vi "ecg_ncs_v1c.vi"() -> ()   [LabVIEW 2016]
uses:
  <instrlib>/niUSRP/niUSRP Timestamp.ctl
  C:/Program Files/National Instruments/LabVIEW 2016/examples/Instrument IO/Serial/support/Serial - Settings.ctl
  <vilib>/Analysis/coordinate.llb/Wrap Angle (array).vi
  <instrlib>/niUSRP/niUSRP Configure Time Start Trigger.vi
  <vilib>/Instr/_visa.llb/VISA Configure Serial Port (Instr).vi
  <instrlib>/niUSRP/niUSRP Write Tx Data (2D CDB).vi
  <instrlib>/niUSRP/niUSRP Fetch Rx Data (2D CDB).vi
  <vilib>/Analysis/3filter.llb/Butterworth Filter (DBL).vi
  <vilib>/measure/NI_MABase.lvlib
  <vilib>/Analysis/NI_AALBase.lvlib
  <vilib>/Analysis/NI_AALPro.lvlib
  <vilib>/Analysis/NI_AAL_Angle.lvlib
panel:
  out "Poor Sensor Quality: \nSensor off":bool
  out "Poor Sensor Quality: \nSensor on":bool
  out "Heart Rate 2":u16[](array[numeric])
  out "Stop Loop":bool
  out "Loop index":i32
  out "size(s)":i32
  in  "Read Count":u32=960
  out "return count":u32
  out "Serial Settings:Number of Bytes at Serial Port":u32
  in  "Serial Settings":T1={"baud rate"=57600, "data bits"=8, "parity"=enum."None", "stop bits"=10, "flow control"=0} {"flow control" items=["None"=0, "XON/XOFF"=1, "RTS/CTS"=2, "DTR/DSR"=4]; "stop bits" items=["1.0"=10, "1.5"=15, "2.0"=20]; "data bits" min=5 max=8 step=1; "baud rate" items=["75"=75, "110"=110, "134"=134, "150"=150, "300"=300, "600"=600, "1200"=1200, "1800"=1800, "2400"=2400, "4800"=4800, "7200"=7200, "9600"=9600, "14400"=14400, "19200"=19200, "28800"=28800, "38400"=38400, "56000"=56000, "57600"=57600, "115200"=115200, "128000"=128000, "230400"=230400]}
  in  "VISA resource name":refnum<visa-resource-name>="bmd101"
  in  "?":enum32{"ECG", "Heart Rate"}(tab)
  out "ECG":i16(graph)
  out "Heart Rate":u8[](graph)
  in  "Stop":bool
  in  "File Name":string="Test"
  in  "order1":i32=5
  in  "Path":path=path "D:/Research/SummerFall17Spring18/CnC/NCS/EcgNcsCorrelation"
  in  "Low-Pass Freq":dbl=200.0 format="%#_13g"
  in  "Sampling Rate":i32=500
  out "Gain":dbl=-15.0
  out "Bandwidth":dbl=56000000.0
  out "Coerced Carrier Frequency":dbl=2000000000.0 format="%#.17g"
  out "Coerced Tx IQ rate":dbl=1000000.0
  out "Coerced Rx IQ rate":dbl=1000000.0
  out "error IO":errorcluster={"status"=FALSE, "code"=-1074118647, "source"=""}
  in  "Rx Number of Samples":i32=20000
  in  "Tab Control 2":enum32{"NI-294x/295x", "NI-2900/2901"}(tab)=enum."NI-2900/2901"
  in  "channel 0 carrier\n frequency [Hz]":dbl=2000000000.0 format="%#_6p"
  in  "Rx carrier frequency [Hz]":dbl=2000000000.0 format="%#_6p"
  in  "Tx carrier frequency [Hz]":dbl=1000000000.0 format="%#_6p"
  in  "Start Trigger Time":T2={"whole seconds"=1, "fractional seconds"=0.0}
  out "Tx Active Antenna":string="TX1"
  in  "Tab Control":T3(tab)
  out "NCS tag Amp":dbl[](graph)=[0.013332788438327721, 0.0131552898712497, 0.012994905519721597, 0.012986271887777701, 0.013075284595455733, 0.013191204808537919, 0.013351894528100879, 0.01345386740636616, 0.013382234051438232, 0.013180163786137358]
  out "NCS tag Phase":dbl[](graph)=[114.08993023907641, 111.82225141412982, 110.02998222947944, 109.41153055749608, 110.12587965469353, 112.16042160734105, 113.81215100166591, 114.51260226782536, 113.6206368361215, 111.46787264294511]
  out "IQ":dbl[][](graph)
  out "Tag Amp":dbl[](graph)
  out "Tag Phase":dbl[](graph)
  out "Tx Waveform Graph":waveform(dbl)[](graph)=[{"t0"=timestamp(0 s since 1904-01-01), "dt"=1e-06, "Y"=array[2000 elements]}, {"t0"=timestamp(0 s since 1904-01-01), "dt"=1e-06, "Y"=array[2000 elements]}]
  in  "Channel 0\nTone Amplitude":dbl=0.707 step=0.05 format="%#.6g"
  in  "Channel 0 \nTone Frequency":dbl=5000.0 format="%#_6p"
  in  "Waveform Size":dbl=2000.0
  in  "Rx Active Antenna":string="RX2"
  in  "Device Name":refnum<k15>="MyB200"
  in  "Tx Gain":dbl=28.0 format="%#_6f"
  in  "Tx IQ Rate":dbl=1000000.0 format="%#_6p"
  in  "Rx Gain":dbl=32.0 format="%#_6f"
  in  "Rx IQ Rate":dbl=1000000.0 format="%#_6p"
  # "Rx Settings"
  # "Tx Settings"
  # "Note that on the NI-2900 and NI-2901, both Rx channels share an LO and both Tx channels share an LO. However, on the NI-294x/295x devices, Rx and Tx of channel 0 share an LO and Rx and Tx of channel 1 share an LO."
  # "This Tx graph should always have end and start tied up since this is being sent in a loop continuously. Otherwise phase jumps will be noticed."
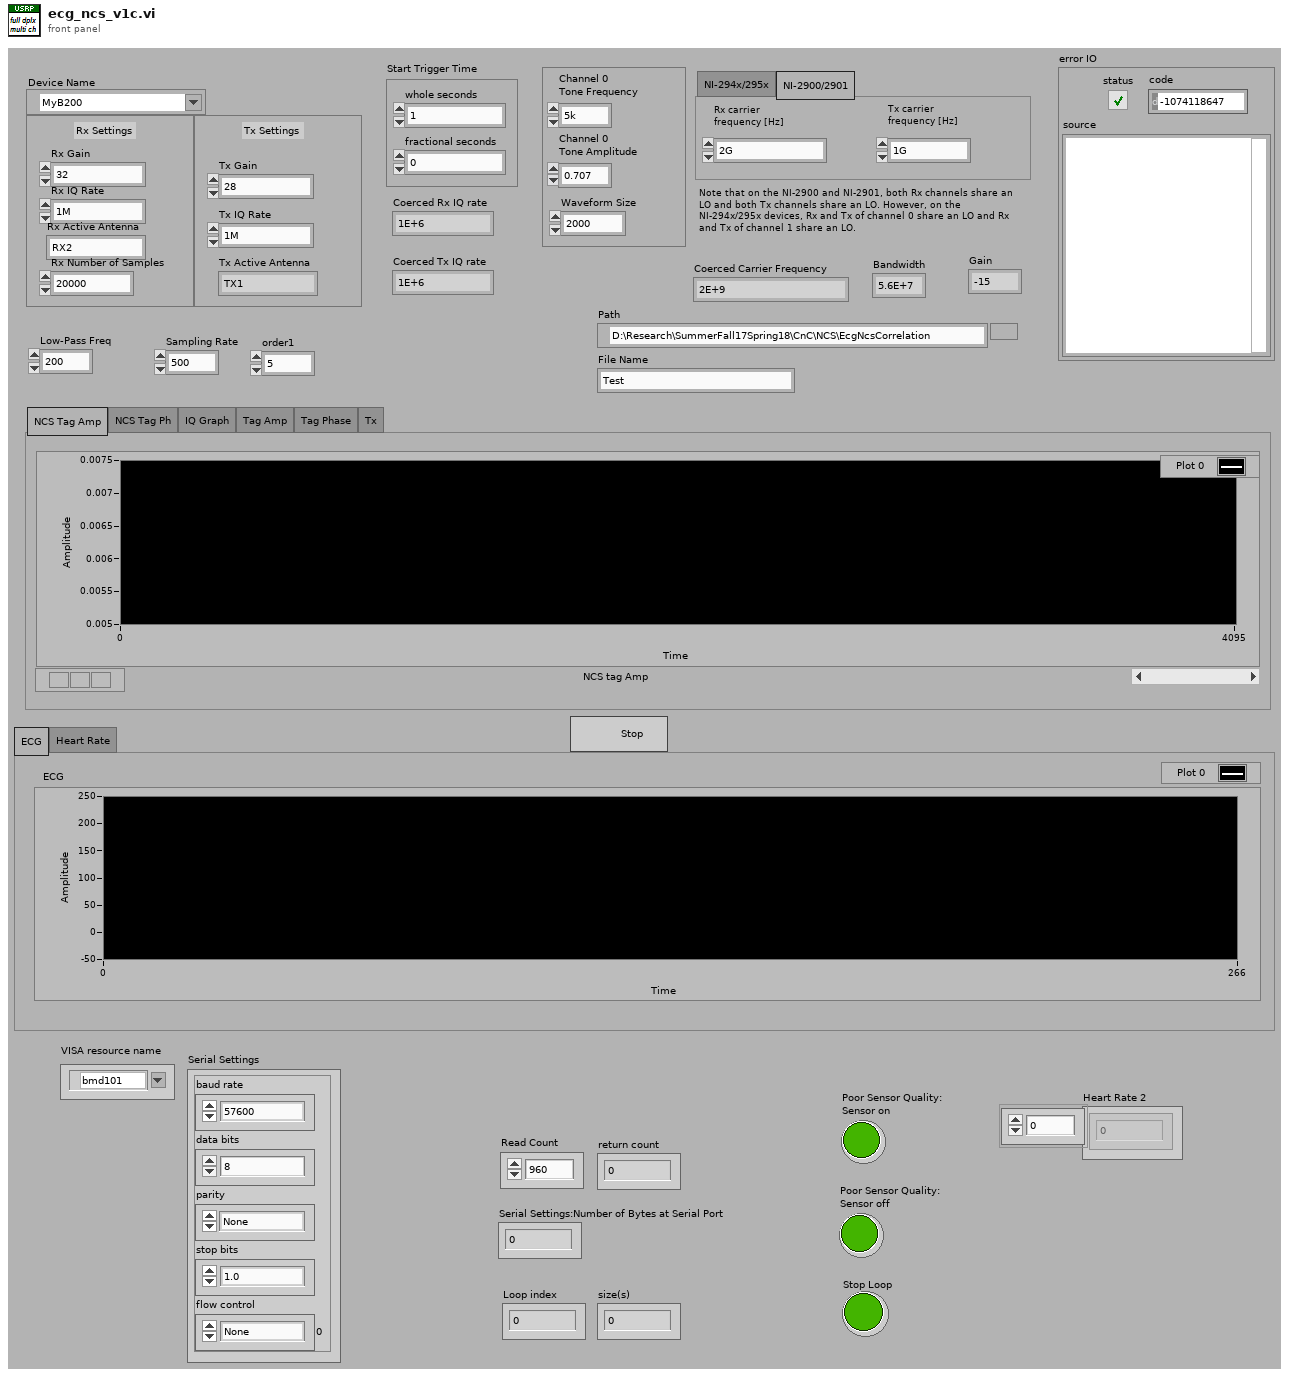
[diagram p1: front panel]
types:
  T1 = typedef "Serial - Settings.ctl" = cluster{"baud rate":u32, "data bits":u16, "parity":enum16{"None", "Odd", "Even", "Mark", "Space"}, "stop bits":u16, "flow control":u16}
  T2 = typedef "niUSRP Timestamp.ctl" = cluster{"whole seconds":u64, "fractional seconds":dbl}
  T3 = enum32{"NCS Tag Amp", "NCS Tag Ph", "IQ Graph", "Tag Amp", "Tag Phase", "Tx"}
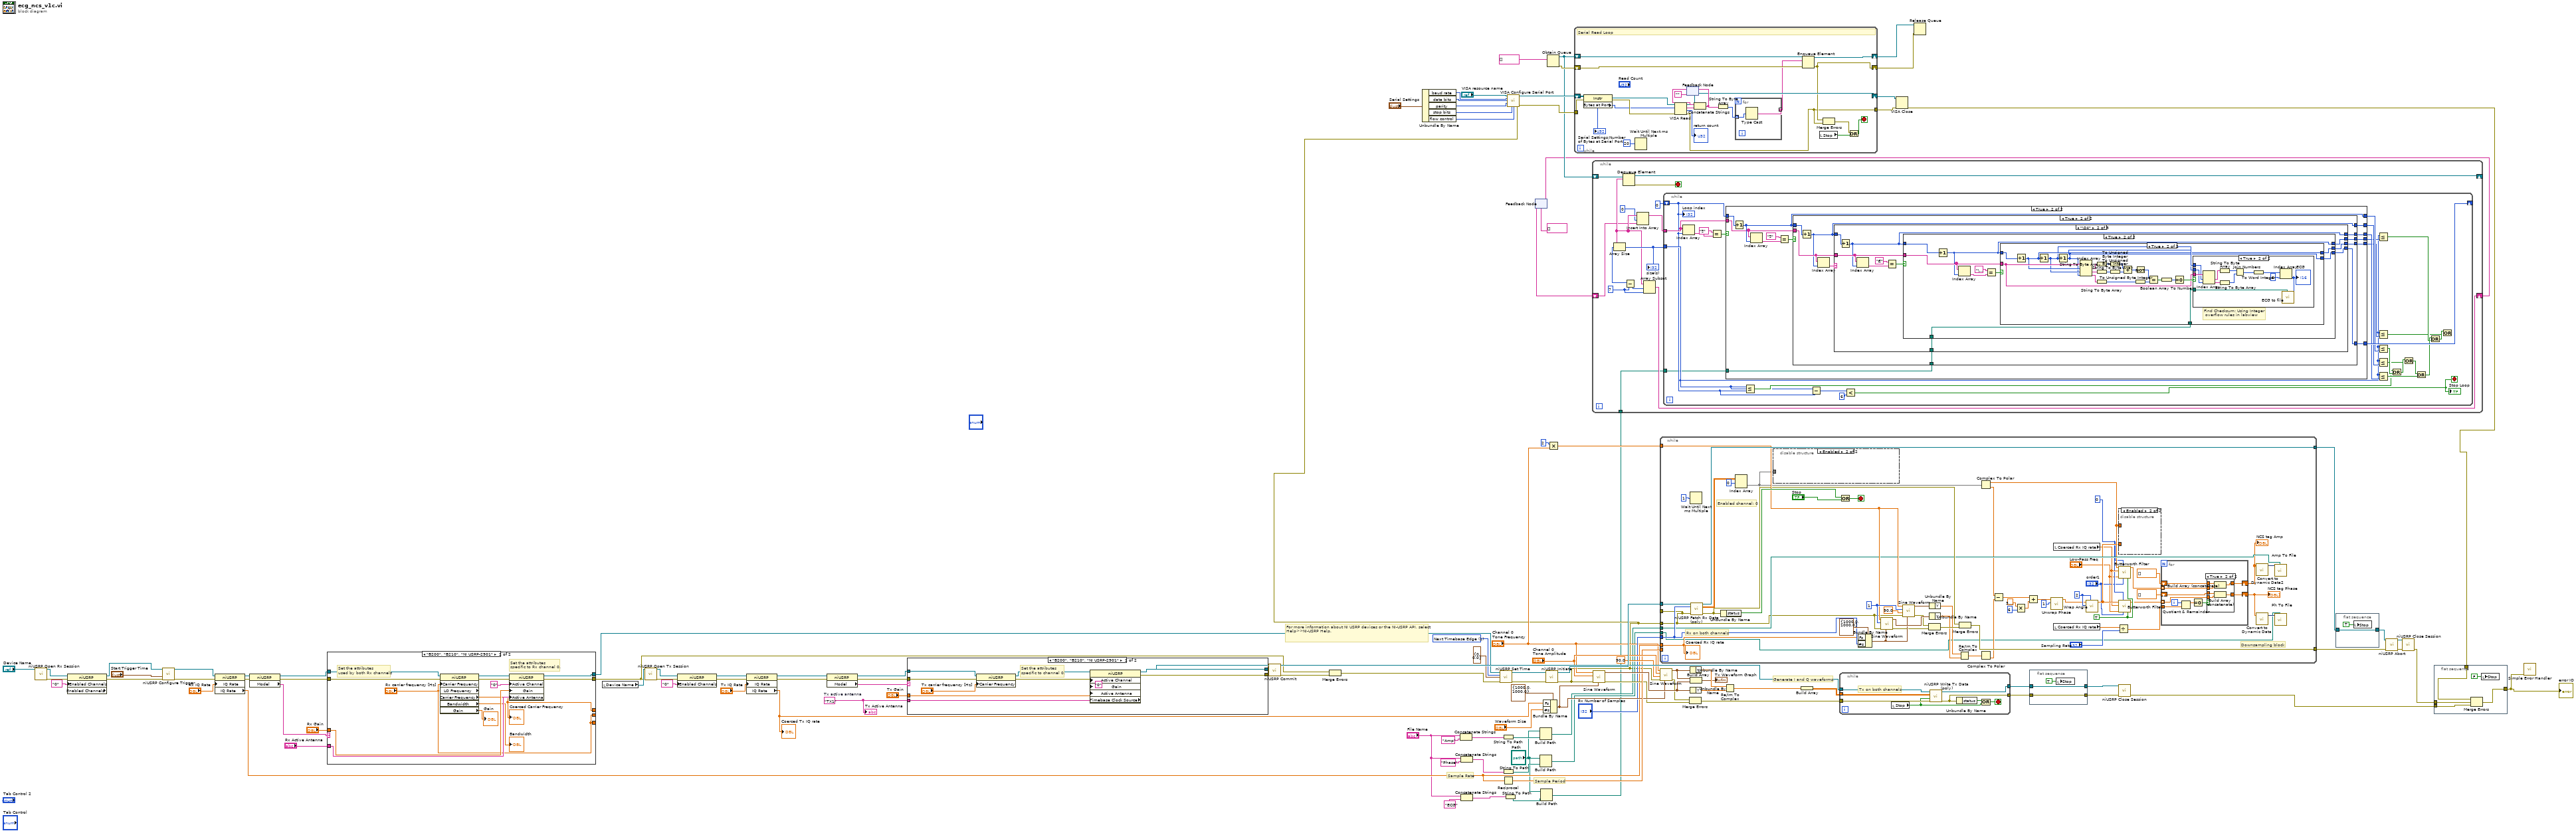
[diagram p0: block diagram]
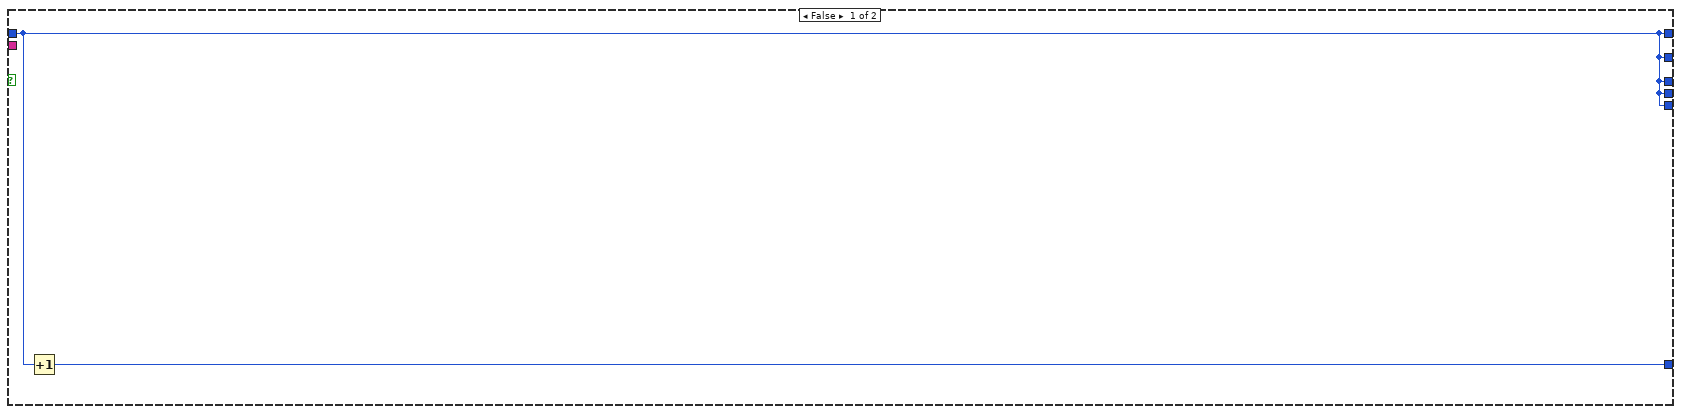
[diagram p2: hidden frame]
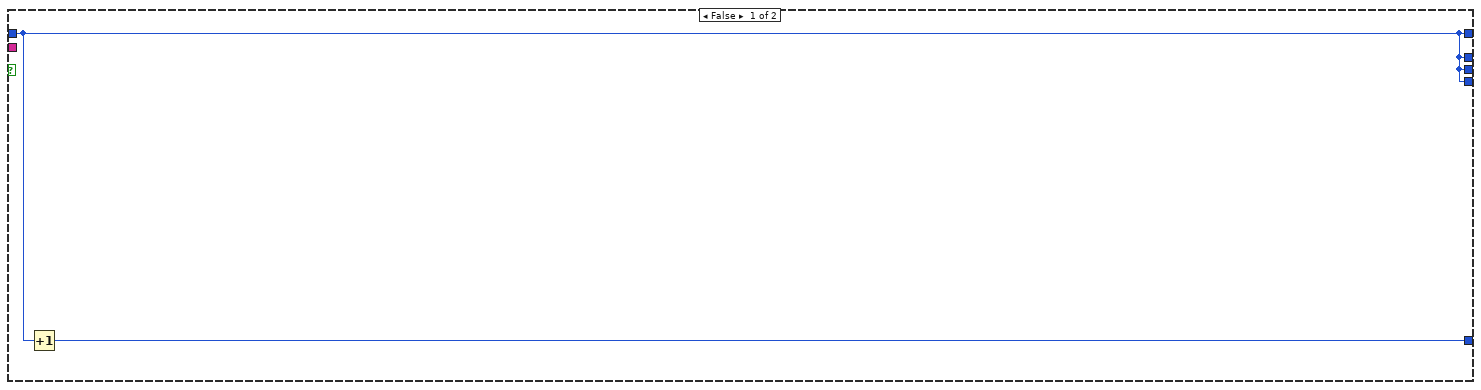
[diagram p3: hidden frame]
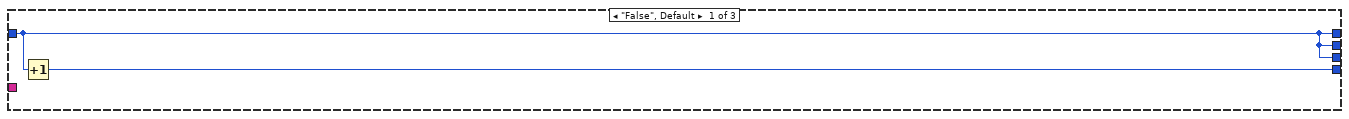
[diagram p4: hidden frame]
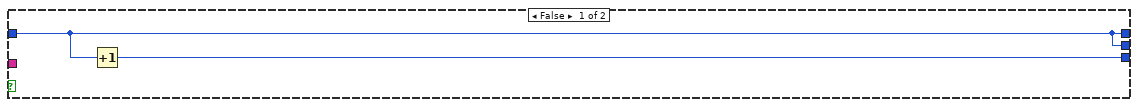
[diagram p5: hidden frame]
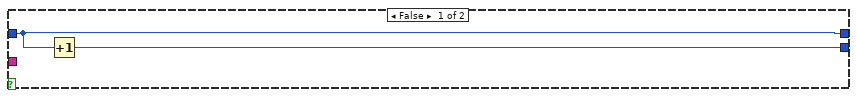
[diagram p6: hidden frame]
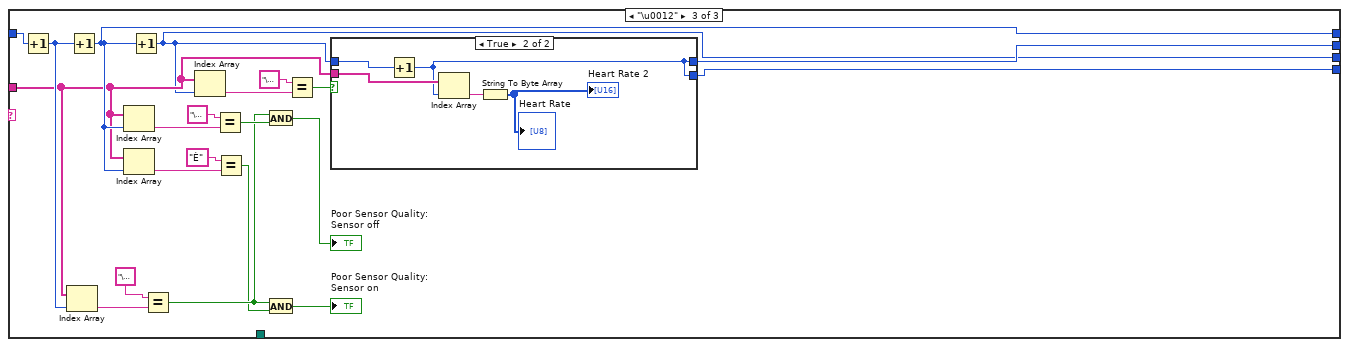
[diagram p8: hidden frame]
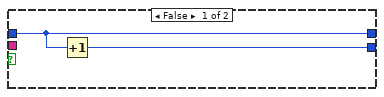
[diagram p9: hidden frame]
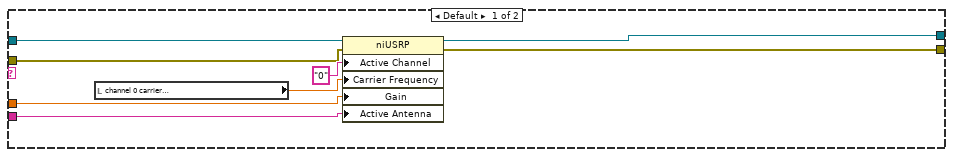
[diagram p10: hidden frame]
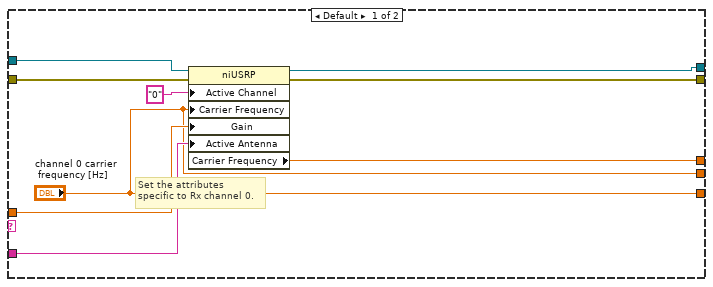
[diagram p11: hidden frame]
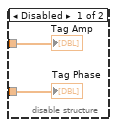
[diagram p12: hidden frame]
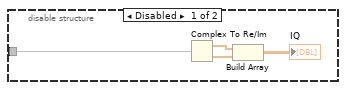
[diagram p13: hidden frame]
diagram:
  w85 = 1 items=["Now", "Next Timebase Edge"] ("apply timestamp")
  w54 = "TX1"  # Tx active antenna
  # "Sample Rate"
  # "Sample Period"
  # "For more information about NI USRP devices or the NI-USRP API, select Help>>NI-USRP Help."
  # "Generate I and Q waveforms."
  n1 = call <instrlib>:"niUSRP Open Rx Session.vi"("device names"="Device Name") -> ("session handle out"=w84:refnum<k15>, "error out"=w83:errorcluster)  [unwired: 13 in]
  n2 = property class="niUSRP" props=["Enabled Channels", "Enabled Channels"](reference=w84, error in=w83, "Enabled Channels"="0" ("Configuration:Enabled Channels")) -> (reference out=w82:refnum<k15>, error out=w81:errorcluster)  [unwired: 1 out]
  n3 = call-poly <instrlib>:"niUSRP Configure Trigger.vi"("session handle"=w82, "start trigger time"="Start Trigger Time", "error in (no error)"=w81) -> ("session handle out"=w78:refnum<k15>, "error out"=w77:errorcluster)  [unwired: 11 in]
  n4 = property class="niUSRP"(reference=w78, error in=w77, "IQ Rate"="Rx IQ Rate") -> (reference out=w74:refnum<k15>, error out=w75:errorcluster, "IQ Rate"=w41:dbl)
  n5 = property class="niUSRP"(reference=w74, error in=w75) -> (reference out=w69:refnum<k15>, error out=w70:errorcluster, "Model"=w71:string)
  n6 = case shown="\"B200\", \"B210\", \"NI USRP-2901\"" w71 {
    tunnel: w70 -> [w120 w130]
    tunnel: w69 -> [w119 w131]
    tunnel: [w116 w127] -> w73
    tunnel: [w115 w126] -> w72
    tunnel: "Rx Gain" -> [w118 w133]
    tunnel: "Rx Active Antenna" -> [w117 w132]
    tunnel: [w113 w122] -> _
    tunnel: ["channel 0 carrier\n frequency [Hz]" "Rx carrier frequency [Hz]"] -> _
    tunnel: ["channel 0 carrier\n frequency [Hz]" "Rx carrier frequency [Hz]"] -> _
    frame Default {
      # "Set the attributes \nspecific to Rx channel 0."
      n7 = property class="niUSRP"(reference=w119, error in=w120, "Active Channel"="0", "Carrier Frequency"="channel 0 carrier\n frequency [Hz]", "Gain"=w118, "Active Antenna"=w117) -> (reference out=w116:refnum<k15>, error out=w115:errorcluster, "Carrier Frequency"=w113:dbl)
    }
    frame "B200", "B210", "NI USRP-2901" {
      # "Set the attributes \nused by both Rx channels"
      # "Set the attributes \nspecific to Rx channel 0."
      n8 = property class="niUSRP" props=["Carrier Frequency", "LO Frequency", "Carrier Frequency", "Bandwidth", "Gain"](reference=w131, error in=w130, "Carrier Frequency"="Rx carrier frequency [Hz]") -> (reference out=w129:refnum<k15>, error out=w128:errorcluster, "Carrier Frequency"=w122:dbl, "Bandwidth"=→"Bandwidth":dbl, "Gain"=→"Gain":dbl)  [unwired: 1 out]
      "Coerced Carrier Frequency" <- w122
      n9 = property class="niUSRP"(reference=w129, error in=w128, "Active Channel"="0", "Gain"=w133, "Active Antenna"=w132) -> (reference out=w127:refnum<k15>, error out=w126:errorcluster)
    }
  }
  n10 = local read "Device Name"() -> (w106:refnum<k15>)
  n11 = call <instrlib>:"niUSRP Open Tx Session.vi"("device names"=w106, "error in (no error)"=w72) -> ("session handle out"=w80:refnum<k15>, "error out"=w79:errorcluster)  [unwired: 12 in]
  n12 = property class="niUSRP"(reference=w80, error in=w79, "Enabled Channels"="0" ("Configuration:Enabled Channels")) -> (reference out=w66:refnum<k15>, error out=w65:errorcluster)
  n13 = property class="niUSRP"(reference=w66, error in=w65, "IQ Rate"="Tx IQ Rate") -> (reference out=w60:refnum<k15>, error out=w61:errorcluster, "IQ Rate"=w58:dbl)
  "Coerced Tx IQ rate" <- w58
  n14 = property class="niUSRP"(reference=w60, error in=w61) -> (reference out=w62:refnum<k15>, error out=w63:errorcluster, "Model"=w59:string)
  n15 = case shown="\"B200\", \"B210\", \"NI USRP-2901\"" w59 {
    tunnel: "Tx Gain" -> [w142 w152]
    tunnel: w54 -> [w140 w150]
    tunnel: [w136 w144] -> w56
    tunnel: [w135 w143] -> w57
    tunnel: w63 -> [w139 w146]
    tunnel: w62 -> [w138 w149]
    frame Default {
      n16 = local read "channel 0 carrier\n frequency [Hz]"() -> (w137:dbl)
      n17 = property class="niUSRP"(reference=w138, error in=w139, "Active Channel"="0", "Carrier Frequency"=w137, "Gain"=w142, "Active Antenna"=w140) -> (reference out=w136:refnum<k15>, error out=w135:errorcluster)
    }
    frame "B200", "B210", "NI USRP-2901" {
      # "Set the attributes \nspecific to channel 0."
      n18 = property class="niUSRP"(reference=w149, error in=w146, "Carrier Frequency"="Tx carrier frequency [Hz]") -> (reference out=w148:refnum<k15>, error out=w147:errorcluster)
      n19 = property class="niUSRP" props=["Active Channel", "Gain", "Active Antenna", "Timebase Clock Source"](reference=w148, error in=w147, "Active Channel"="0", "Gain"=w152, "Active Antenna"=w150) -> (reference out=w144:refnum<k15>, error out=w143:errorcluster)  [unwired: 1 out]
    }
  }
  n20 = call <instrlib>:"niUSRP Commit.vi"("session handle"=w56, "error in (no error)"=w57) -> ("session handle out"=w108:refnum<k15>, "error out"=w109:errorcluster)  [unwired: 12 in]
  n21 = Merge Errors(w72, w109) -> (w87:errorcluster)
  n22 = Unbundle By Name("Serial Settings") -> ("baud rate"=w26:u32, "data bits"=w25:u16, "parity"=w24:enum16{"None", "Odd", "Even", "Mark", "Space"}, "stop bits"=w23:u16, "flow control"=w22:u16)
  n23 = Concatenate Strings("File Name", "Amp") -> (w34:string)
  n24 = Concatenate Strings("File Name", "Phase") -> (w31:string)
  n25 = Concatenate Strings("File Name", "ECG") -> (w4:string)
  n26 = call <instrlib>:"niUSRP Set Time.vi"("session handle"=w73, "apply timestamp"=w85, "timestamp"=T2 {"whole seconds"=0, "fractional seconds"=0.0}, "error in (no error)"=w87) -> ("session handle out"=w89:refnum<k15>, "error out"=w88:errorcluster)  [unwired: 10 in]
  n27 = String To Path(string=w34) -> (path=w33:path)
  n28 = String To Path(string=w31) -> (path=w30:path)
  n29 = Reciprocal(x=w41) -> (1/x=w92:dbl)
  n30 = String To Path(string=w4) -> (path=w3:path)
  n31 = feedback #1(string[] []) -> (w10:string[])
  n32 = Build Path(base path="Path", name or relative path=w33) -> (appended path=w36:path)
  n33 = Build Path(base path="Path", name or relative path=w30) -> (appended path=w29:path)
  n34 = Build Path(base path="Path", name or relative path=w3) -> (appended path=w6:path)
  n35 = Bundle By Name(cluster=cluster{"Fs":dbl, "#s":dbl} {"Fs"=1000.0, "#s"=1000.0} ("sampling info"), "Fs"=w58, "#s"="Waveform Size") -> (w91:cluster{"Fs":dbl, "#s":dbl})
  n36 = call <instrlib>:"niUSRP Initiate.vi"("session handle"=w89, "error in (no error)"=w88) -> ("session handle out"=w112:refnum<k15>, "error out"=w7:errorcluster)  [unwired: 12 in]
  n37 = call-poly "VISA Configure Serial Port"("VISA resource name"="VISA resource name", "baud rate (9600)"=w26, "data bits (8)"=w25, "parity (0:none)"=w24, "error in (no error)"=w7, "stop bits (10: 1 bit)"=w23, "flow control (0:none)"=w22) -> ("VISA resource name out"=w18:refnum<visa-resource-name>, "error out"=w17:errorcluster)  [unwired: 3 in, 4 out]
  n38 = Obtain Queue(element data type=string[] []) -> (queue out=w12:refnum<queue>, error out=w14:errorcluster)  [unwired: 4 in, 1 out]
  n39 = Multiply(x=2, y="Channel 0 \nTone Frequency") -> (x*y=w38:dbl)
  n40 = while {
    shift-right: [w167] -> w19
    shift-left: w18 -> [w158]
    tunnel: w17 -> [w156]
    tunnel: [w160] -> w20
    shift-right: [w161] -> w16
    shift-left: w14 -> [w165]
    shift-right: [w162] -> w13
    shift-left: w12 -> [w163]
    stop <- w174 stop-if-true
    # "Serial Read Loop"
    n41 = property class="Instr"(reference=w158, error in=w156) -> (reference out=w157:refnum<visa-resource-name>, error out=w155:errorcluster, "Bytes at Port"=w154:u32)
    "Serial Settings:Number of Bytes at Serial Port" <- w154
    n42 = Wait Until Next ms Multiple(millisecond multiple=u32 20 ("milliseconds to wait")) -> ()  [unwired: 1 out]
    n43 = VISA Read(VISA resource name=w157, byte count=w154, error in (no error)=w155) -> (VISA resource name out=w167:refnum<visa-resource-name>, read buffer=w172:string, return count=→"return count":u32, error out=w160:errorcluster)
    n44 = feedback #2("") -> (w171:string)
    n45 = Concatenate Strings(w171, w172) -> (w169:string)
    n46 = feedback-in #2(w169) -> ()
    n47 = String To Byte Array(string=w169) -> (unsigned byte array=w166:u8[])
    n48 = for {
      tunnel: w166 -> [w176] mode=indexing
      tunnel: [w175] -> w164 mode=indexing
      n49 = Type Cast(x=w176) -> (*(type *) &x=w175:string)  [unwired: 1 in]
    }
    n50 = Enqueue Element(queue=w163, element=w164, error in (no error)=w165) -> (queue out=w162:refnum<queue>, error out=w161:errorcluster)  [unwired: 1 in, 1 out]
    n51 = local read "Stop"() -> (w153:bool)
    n52 = Merge Errors(w161, w160) -> (w159:errorcluster)
    n53 = Or(x=w159, y=w153) -> (x .or. y?=w174:bool)
  }
  n54 = while {
    shift-right: [w187] -> _
    shift-left: w12 -> [w188]
    shift-right: [w180] -> w11
    shift-left: w10 -> [w178]
    tunnel: w6 -> [w177]
    stop <- w186 stop-if-true
    w183 = 7
    n55 = Dequeue Element(queue=w188) -> (queue out=w187:refnum<queue>, element=w181:string[], error out=w186:errorcluster)  [unwired: 2 in, 1 out]
    n56 = Array Size(array=w181) -> (size(s)=w185:i32)
    "size(s)" <- w185
    n57 = Subtract(x=w185, y=w183) -> (x-y=w184:i32)
    n58 = Insert Into Array(array=w181, index=0, new element=w178) -> (w182:string[])
    n59 = Array Subset(array=w181, index=w184, length=w183) -> (w180:string[])
    n60 = while {
      tunnel: w182 -> [w211]
      shift-right: [w215] -> _
      shift-left: 0 -> [w194]
      tunnel: w185 -> [w195]
      tunnel: w177 -> [w190]
      stop <- w191 stop-if-true
      n61 = Index Array(array=w211, index=w194) -> (element=w214:string)
      n62 = Equal?(x="ª", y=w214) -> (x = y?=w212:bool)
      n63 = case shown="True" w212 {
        tunnel: w194 -> [w216 w227]
        tunnel: [w217 w225] -> w215
        tunnel: w211 -> [_ w219]
        tunnel: [w216 w224] -> w210
        tunnel: [w216 w223] -> w208
        tunnel: [w216 w222] -> w205
        tunnel: [w216 w221] -> w202
        tunnel: [w216 w220] -> w199
        tunnel: w190 -> [_ w218]
        frame False {
          n64 = Increment(x=w216) -> (x+1=w217:i32)
        }
        frame True {
          n65 = Increment(x=w227) -> (x+1=w224:i32)
          n66 = Index Array(array=w219, index=w224) -> (element=w229:string)
          n67 = Equal?(x="ª", y=w229) -> (x = y?=w226:bool)
          n68 = case shown="True" w226 {
            tunnel: w224 -> [w230 w234]
            tunnel: [w231 w240] -> w225
            tunnel: w219 -> [_ w239]
            tunnel: [w230 w235] -> w223
            tunnel: [w230 w238] -> w222
            tunnel: [w230 w237] -> w221
            tunnel: [w230 w236] -> w220
            tunnel: w218 -> [_ w232]
            frame False {
              n69 = Increment(x=w230) -> (x+1=w231:i32)
            }
            frame True {
              n70 = Increment(x=w234) -> (x+1=w235:i32)
              n71 = Index Array(array=w239, index=w235) -> (element=w233:string)
              n72 = case shown="\"\\04\"" w233 {
                tunnel: w235 -> [w241 w249 w317]
                tunnel: [w242 w248 w299] -> w240
                tunnel: w239 -> [_ w247 w301]
                tunnel: [w241 w246 w303] -> w238
                tunnel: [w241 w245 w300] -> w237
                tunnel: [w241 w244 w298] -> w236
                tunnel: w232 -> [_ w243 _]
                frame "False", Default {
                  n73 = Increment(x=w241) -> (x+1=w242:i32)
                }
                frame "\u0004" {
                  n74 = Increment(x=w249) -> (x+1=w246:i32)
                  n75 = Index Array(array=w247, index=w246) -> (element=w250:string)
                  n76 = Equal?(x="€", y=w250) -> (x = y?=w251:bool)
                  n77 = case shown="True" w251 {
                    tunnel: w246 -> [w253 w260]
                    tunnel: [w254 w259] -> w248
                    tunnel: w247 -> [_ w258]
                    tunnel: [w253 w257] -> w245
                    tunnel: [w253 w256] -> w244
                    tunnel: w243 -> [_ w255]
                    frame False {
                      n78 = Increment(x=w253) -> (x+1=w254:i32)
                    }
                    frame True {
                      n79 = Increment(x=w260) -> (x+1=w257:i32)
                      n80 = Index Array(array=w258, index=w257) -> (element=w261:string)
                      n81 = Equal?(x="\u0002", y=w261) -> (x = y?=w262:bool)
                      n82 = case shown="True" w262 {
                        tunnel: w257 -> [w264 w270]
                        tunnel: [w265 w267] -> w259
                        tunnel: w258 -> [_ w271]
                        tunnel: [w264 w267] -> w256
                        tunnel: w255 -> [_ w266]
                        frame False {
                          n83 = Increment(x=w264) -> (x+1=w265:i32)
                        }
                        frame True {
                          # "Find Checksum: Using Integer\n overflow rules in labview"
                          n84 = Increment(x=w270) -> (x+1=w269:i32)
                          n85 = Increment(x=w269) -> (x+1=w268:i32)
                          n86 = Increment(x=w268) -> (x+1=w267:i32)
                          n87 = Index Array(array=w271, index #1=w269, index #2=w268, index #3=w267) -> (element #1=w285:string, element #2=w284:string, element #3=w278:string)
                          n88 = String To Byte Array(string=w285) -> (unsigned byte array=w283:u8[])
                          n89 = String To Byte Array(string=w284) -> (unsigned byte array=w282:u8[])
                          n90 = String To Byte Array(string=w278) -> (unsigned byte array=w277:u8[])
                          n91 = To Unsigned Byte Integer(number=w283) -> (unsigned 8bit integer=w281:u8[])
                          n92 = To Unsigned Byte Integer(number=w282) -> (unsigned 8bit integer=w280:u8[])
                          n93 = Add(x=w281, y=w280) -> (x+y=w279:u8[])
                          n94 = Not(x=w279) -> (.not. x?=w276:u8[])
                          n95 = To Unsigned Byte Integer(number=w277) -> (unsigned 8bit integer=w275:u8[])
                          n96 = Equal?(x=w276, y=w275) -> (x = y?=w274:bool[])
                          n97 = Boolean Array To Number(Boolean array=w274) -> (number=w273:u32)
                          n98 = Equal To 0?(x=w273) -> (x = 0?=w272:bool)
                          n99 = case shown="True" w272 {
                            tunnel: w271 -> [_ w297]
                            tunnel: w269 -> [_ w291]
                            tunnel: w268 -> [_ w290]
                            tunnel: w266 -> [_ w286]
                            frame False {
                            }
                            frame True {
                              n100 = Index Array(array=w297, index #1=w291, index #2=w290) -> (element #1=w296:string, element #2=w295:string)
                              n101 = String To Byte Array(string=w296) -> (unsigned byte array=w294:u8[])
                              n102 = String To Byte Array(string=w295) -> (unsigned byte array=w293:u8[])
                              n103 = Join Numbers(hi=w294, lo=w293) -> ((hi.lo)=w292:u16[])
                              n104 = To Word Integer(number=w292) -> (16bit integer=w289:i16[])
                              n105 = Index Array(array=w289, index=0) -> (element=w287:i16)
                              "ECG" <- w287
                              n106 = call "ECG to file"("Signals"=w287, "Filename"=w286) -> ()  [unwired: 15 in, 3 out]
                            }
                          }
                        }
                      }
                    }
                  }
                }
                frame "\u0012" {
                  n107 = Increment(x=w317) -> (x+1=w313:i32)
                  n108 = Index Array(array=w301, index=w313) -> (element=w316:string)
                  n109 = Increment(x=w313) -> (x+1=w303:i32)
                  n110 = Index Array(array=w301, index=w303) -> (element=w314:string)
                  n111 = Index Array(array=w301, index=w303) -> (element=w311:string)
                  n112 = Increment(x=w303) -> (x+1=w298:i32)
                  n113 = Equal?(x="\u0002", y=w316) -> (x = y?=w308:bool)
                  n114 = Index Array(array=w301, index=w298) -> (element=w304:string)
                  n115 = Equal?(x="\u0000", y=w314) -> (x = y?=w310:bool)
                  n116 = Equal?(x="È", y=w311) -> (x = y?=w307:bool)
                  n117 = And(x=w308, y=w310) -> (x .and. y?=→"Poor Sensor Quality: \nSensor off":bool)
                  n118 = And(x=w308, y=w307) -> (x .and. y?=→"Poor Sensor Quality: \nSensor on":bool)
                  n119 = Equal?(x="\u0003", y=w304) -> (x = y?=w302:bool)
                  n120 = case shown="True" w302 {
                    tunnel: w298 -> [w319 w325]
                    tunnel: w301 -> [_ w324]
                    tunnel: [w319 w323] -> w300
                    tunnel: [w320 w323] -> w299
                    frame False {
                      n121 = Increment(x=w319) -> (x+1=w320:i32)
                    }
                    frame True {
                      n122 = Increment(x=w325) -> (x+1=w323:i32)
                      n123 = Index Array(array=w324, index=w323) -> (element=w322:string)
                      n124 = String To Byte Array(string=w322) -> (unsigned byte array=→"Heart Rate 2" →"Heart Rate":u8[])
                    }
                  }
                }
              }
            }
          }
        }
      }
      n125 = Less Or Equal?(x=w195, y=w194) -> (x <= y?=w196:bool)
      n126 = Subtract(x=w195, y=w194) -> (x-y=w193:i32)
      n127 = Less?(x=w193, y=6) -> (x < y?=w191:bool)
      "Stop Loop" <- w191
      n128 = Less Or Equal?(x=w195, y=w202) -> (x <= y?=w200:bool)
      n129 = Less Or Equal?(x=w195, y=w199) -> (x <= y?=w197:bool)
      n130 = Less Or Equal?(x=w195, y=w210) -> (x <= y?=w209:bool)
      n131 = Less Or Equal?(x=w195, y=w208) -> (x <= y?=w206:bool)
      n132 = Less Or Equal?(x=w195, y=w205) -> (x <= y?=w203:bool)
      n133 = Or(x=w196, y=w209) -> (x .or. y?=w207:bool)
      n134 = Or(x=w207, y=w206) -> (x .or. y?=w204:bool)
      n135 = Or(x=w204, y=w203) -> (x .or. y?=w201:bool)
      n136 = Or(x=w201, y=w200) -> (x .or. y?=w198:bool)
      n137 = Or(x=w198, y=w197) -> ()  [unwired: 1 out]
      "Loop index" <- w194
    }
  }
  n138 = feedback-in #1(w11) -> ()
  n139 = call <vilib>:"Sine Waveform.vi"("sampling info"=w91, "error in (no error)"=w7, "amplitude"="Channel 0\nTone Amplitude", "frequency"="Channel 0 \nTone Frequency") -> ("error out"=w53:errorcluster, "signal out"=w101:waveform(dbl))  [unwired: 6 in]
  n140 = while {
    tunnel: w112 -> [w382]
    tunnel: w7 -> [w327]
    tunnel: [w381] -> w47
    tunnel: w92 -> [_]
    tunnel: "Rx Number of Samples" -> [w377]
    tunnel: w41 -> [w368]
    tunnel: w38 -> [w369]
    tunnel: [w358] -> w37
    tunnel: w36 -> [w357]
    tunnel: w29 -> [w332]
    tunnel: [w327] -> _
    stop <- w359 stop-if-true
    w344 = 2 ("y")
    w337 = TRUE
    w339 = 0
    w375 = 1
    # "Downsampling block"
    # "Enabled channel: 0"
    # "Rx on both channels"
    n141 = Wait Until Next ms Multiple(millisecond multiple=u32 1 ("milliseconds to wait")) -> ()  [unwired: 1 out]
    n142 = call-poly <instrlib>:"niUSRP Fetch Rx Data (poly).vi"("session handle"=w382, "number of samples"=w377, "error in (no error)"=w327) -> ("session handle out"=w381:refnum<k15>, "data"=w366:cdb[][], "error out"=w363:errorcluster)  [unwired: 9 in, 1 out]
    n143 = Unbundle By Name(w363) -> ("status"=w380:bool)
    n144 = Index Array(array=w366, index (row)=0 ("y")) -> (element=w365:cdb[])  [unwired: 1 in]
    n145 = disable-structure shown="Enabled" {
      disable-tunnel: w365 -> [w385 _]
      frame Disabled {
        n146 = Complex To Re/Im(x + iy=w385) -> (x=w388:dbl[], y=w387:dbl[])
        n147 = Build Array(w388, w387) -> (→"IQ":dbl[][])
      }
      frame Enabled {
      }
    }
    n148 = Or(x=w380, y="Stop") -> (x .or. y?=w359:bool)
    n149 = Bundle By Name(cluster=cluster{"Fs":dbl, "#s":dbl} {"Fs"=1000.0, "#s"=1000.0} ("sampling info"), "Fs"=w368, "#s"=w377) -> (w374:cluster{"Fs":dbl, "#s":dbl})
    n150 = call <vilib>:"Sine Waveform.vi"("sampling info"=w374, "error in (no error)"=w327, "amplitude"=w375, "frequency"=w369) -> ("error out"=w373:errorcluster, "signal out"=w378:waveform(dbl))  [unwired: 6 in]
    n151 = call <vilib>:"Sine Waveform.vi"("sampling info"=w374, "error in (no error)"=w327, "phase"=90.0, "amplitude"=w375, "frequency"=w369) -> ("error out"=w372:errorcluster, "signal out"=w370:waveform(dbl))  [unwired: 5 in]
    n152 = Merge Errors(w372, w373) -> (w371:errorcluster)
    n153 = Unbundle By Name(w370) -> ("Y"=w354:dbl[])
    n154 = Unbundle By Name(w378) -> ("Y"=w353:dbl[])
    n155 = Re/Im To Complex(1:w353, 2:w354) -> (0:w347:cdb[])
    n156 = Merge Errors(w363, w371) -> (w358:errorcluster)
    n157 = Complex To Polar(r * e^(i*theta)=w365) -> (r=w356:dbl[], theta=w342:dbl[])
    n158 = Complex To Polar(r * e^(i*theta)=w347) -> (theta=w348:dbl[])  [unwired: 1 out]
    n159 = Subtract(x=w342, y=w348) -> (x-y=w346:dbl[])
    n160 = Multiply(x=3.141592653589793, y=6) -> (x*y=w349:dbl)
    n161 = Add(x=w346, y=w349) -> (x+y=w345:dbl[])
    n162 = call <vilib>:"Unwrap Phase.vi"("phase unit"=1 ("y"), "Phase"=w345) -> ("Unwrapped Phase"=w343:dbl[])  [unwired: 8 in, 1 out]
    n163 = local read "Coerced Rx IQ rate"() -> (w340:dbl)
    n164 = local read "Coerced Rx IQ rate"() -> (w362:dbl)
    n165 = call-poly <vilib>:"Wrap Angle.vi"("angle units"=w344, "angle range"=w344, "Angle In"=w343) -> ("Angle Out"=w341:dbl[])  [unwired: 7 in, 1 out]
    n166 = Divide(x=w362, y="Sampling Rate") -> (x/y=w360:dbl)
    n167 = disable-structure shown="Enabled" {
      disable-tunnel: w356 -> [w384 _]
      disable-tunnel: w341 -> [w383 _]
      frame Disabled {
        "Tag Amp" <- w384
        "Tag Phase" <- w383
      }
      frame Enabled {
      }
    }
    n168 = call-poly <vilib>:"Butterworth Filter.vi"("init/cont (init:F)"=w337, "order"="order1", "filter type"=w339, "low cutoff freq: fl"="Low-Pass Freq", "sampling freq: fs"=w340, "X"=w356) -> ("Filtered X"=w355:dbl[])  [unwired: 2 in, 1 out]
    n169 = call-poly <vilib>:"Butterworth Filter.vi"("init/cont (init:F)"=w337, "order"="order1", "filter type"=w339, "low cutoff freq: fl"="Low-Pass Freq", "sampling freq: fs"=w340, "X"=w341) -> ("Filtered X"=w335:dbl[])  [unwired: 2 in, 1 out]
    n170 = for {
      tunnel: w355 -> [w398] mode=indexing
      shift-right: [w396] -> w330
      shift-left: dbl[] [] -> [w397]
      tunnel: w360 -> [w392]
      shift-right: [w390] -> w333
      shift-left: dbl[] [] -> [w391]
      tunnel: w335 -> [w389] mode=indexing
      i -> [w395]
      n171 = Quotient & Remainder(x=w395, y=w392) -> (x-y*floor(x/y)=w393:dbl)  [unwired: 1 out]
      n172 = Equal To 0?(x=w393) -> (x = 0?=w394:bool)
      n173 = case shown="True" w394 {
        tunnel: w398 -> [_ w406]
        tunnel: w397 -> [w400 w405]
        tunnel: [w400 w404] -> w396
        tunnel: w391 -> [w399 w403]
        tunnel: [w399 w402] -> w390
        tunnel: w389 -> [_ w401]
        frame False {
        }
        frame True {
          n174 = Build Array (concatenate)(w405, w406) -> (w404:dbl[])
          n175 = Build Array (concatenate)(w403, w401) -> (w402:dbl[])
        }
      }
    }
    "NCS tag Amp" <- w330
    "NCS tag Phase" <- w333
    n176 = call "Convert to Dynamic Data2"("Array"=w330) -> ("Dynamic Data Type"=w329:dynamicdata)  [unwired: 3 in]
    n177 = call "Convert to Dynamic Data"("Array"=w333) -> ("Dynamic Data Type"=w334:dynamicdata)  [unwired: 3 in]
    n178 = call "Amp To File"("Signals"=w329, "Filename"=w357) -> ()  [unwired: 15 in, 3 out]
    n179 = call "Ph To File"("Signals"=w334, "Filename"=w332) -> ()  [unwired: 15 in, 3 out]
    "Coerced Rx IQ rate" <- w368
  }
  n180 = call <vilib>:"Sine Waveform.vi"("sampling info"=w91, "error in (no error)"=w7, "phase"=90.0, "amplitude"="Channel 0\nTone Amplitude", "frequency"="Channel 0 \nTone Frequency") -> ("error out"=w52:errorcluster, "signal out"=w100:waveform(dbl))  [unwired: 5 in]
  n181 = Merge Errors(w52, w53) -> (w51:errorcluster)
  n182 = Unbundle By Name(w100) -> ("Y"=w99:dbl[])
  n183 = Build Array(w100, w101) -> (→"Tx Waveform Graph":waveform(dbl)[])
  n184 = Unbundle By Name(w101) -> ("Y"=w98:dbl[])
  n185 = Re/Im To Complex(1:w98, 2:w99) -> (0:w94:cdb[])
  n186 = Build Array(w94) -> (w93:cdb[][])
  n187 = while {
    tunnel: w108 -> [w414]
    tunnel: w51 -> [w413]
    tunnel: [w411] -> w50
    tunnel: [w409] -> w45
    tunnel: w93 -> [w408]
    stop <- w410 stop-if-true
    # "Tx on both channels"
    n188 = local read "Stop"() -> (w407:bool)
    n189 = call-poly <instrlib>:"niUSRP Write Tx Data (poly).vi"("session handle"=w414, "data"=w408, "end of data?"=w407, "error in (no error)"=w413) -> ("session handle out"=w409:refnum<k15>, "error out"=w411:errorcluster)  [unwired: 10 in]
    n190 = Unbundle By Name(w411) -> ("status"=w412:bool)
    n191 = Compound Arithmetic op=OR(w412, w407) -> (w410:bool)
  }
  n192 = VISA Close(VISA resource name=w19, error in (no error)=w20) -> (error out=w8:errorcluster)
  n193 = Release Queue(queue=w13, error in (no error)=w16) -> ()  [unwired: 1 in, 3 out]
  n194 = flat-sequence {
    tunnel: [w416] -> w49
    tunnel: w50 -> [w416]
    tunnel: [w415] -> w46
    tunnel: w45 -> [w415]
    frame #0 {
      n195 = local write "Stop"(TRUE ("STOP")) -> ()
    }
  }
  n196 = call <instrlib>:"niUSRP Close Session.vi"("session handle"=w46, "error in (no error)"=w49) -> ("error out"=w44:errorcluster)  [unwired: 13 in]
  n197 = flat-sequence {
    tunnel: [w418] -> w48
    tunnel: w47 -> [w418]
    frame #0 {
      n198 = local write "Stop"(TRUE ("STOP")) -> ()
    }
  }
  n199 = call <instrlib>:"niUSRP Abort.vi"("session handle"=w48, "error in (no error)"=w37) -> ("session handle out"=w105:refnum<k15>, "error out"=w104:errorcluster)  [unwired: 12 in]
  n200 = call <instrlib>:"niUSRP Close Session.vi"("session handle"=w105, "error in (no error)"=w104) -> ("error out"=w42:errorcluster)  [unwired: 13 in]
  n201 = flat-sequence {
    tunnel: w44 -> [w423]
    tunnel: [w422] -> w28
    tunnel: w42 -> [w421]
    tunnel: w8 -> [w420]
    frame #0 {
      n202 = Merge Errors(w420, w421, w423) -> (w422:errorcluster)
      n203 = local write "Stop"(FALSE ("STOP")) -> ()
    }
  }
  n204 = call <vilib>:"Simple Error Handler.vi"("error in (no error)"=w28) -> ()  [unwired: 1 in, 8 out]
  "Tx Active Antenna" <- w54
  "error IO" <- w28
